vi "Create.vi"(8 "error in (no error)":errorcluster, 10 "Report Path":path) -> (0 "error out":errorcluster, 3 "XML Report":refnum<class "XML Report.lvclass">)   [LabVIEW 2020, in "XML Report.lvclass"]
uses:
  XML Report.lvclass
  XML Report.lvclass/XML Report.ctl
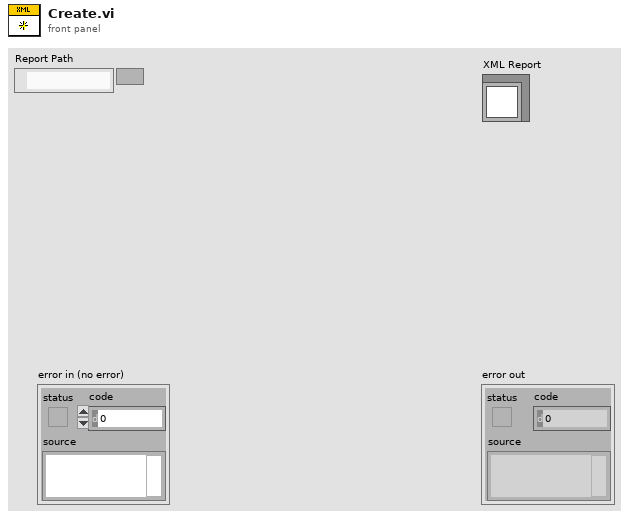
[diagram p1: front panel]
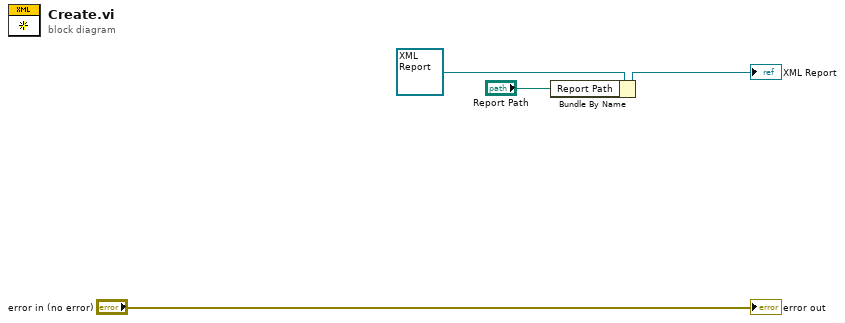
[diagram p0: block diagram]
diagram:
  n1 = Bundle By Name(cluster=refnum<class "XML Report.lvclass"> refnum ("XML Report"), "Report Path"="Report Path") -> (→"XML Report":refnum<class "XML Report.lvclass">)
  "error out" <- "error in (no error)"
